vi "StopMotion.vi"(8 "error in (no error)":errorcluster, 11 "UI ExecutionCtrls in":refnum<class "UI ExecutionCtrls.lvclass">) -> (0 "error out":errorcluster, 3 "UI ExecutionCtrls out":refnum<class "UI ExecutionCtrls.lvclass">)   [LabVIEW 2018, in "UI ExecutionCtrls.lvclass"]
uses:
  UI ExecutionCtrls.lvclass
  UI ExecutionCtrls.lvclass/UI ExecutionCtrls.ctl
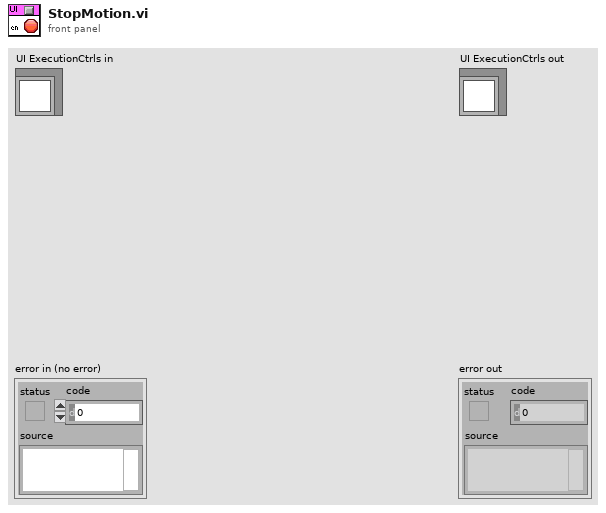
[diagram p1: front panel]
types:
  T1 = enum8{"Enabled", "Disabled", "Disabled and Grayed Out"}
  T2 = typedef "MotionExecutionCtrlRefs.ctl" = cluster{"MoveAllAbsolute":refnum<vi>, "Move to Pos.":refnum<vi>, "HomeAll":refnum<vi>, "FindHomeAll":refnum<vi>, "X Jog Pos.":refnum<vi>, "X Jog Neg.":refnum<vi>, "Y Jog Pos.":refnum<vi>, "Y Jog Neg. ":refnum<vi>, "Z Jog Pos.":refnum<vi>, "Z Jog Neg.":refnum<vi>, "T Jog Pos.":refnum<vi>, "T Jog Neg.":refnum<vi>, "X Home Button":refnum<vi>, "Y Home Button":refnum<vi>, "Z Home Button":refnum<vi>, "T Home Button":refnum<vi>}
  T3 = typedef "mmWaveMotionCrtlRefs.ctl" = cluster{"BS3 Jog Neg. 2":refnum<vi>, "BS3 Jog Pos. 2":refnum<vi>, "BS3 Home Button 2":refnum<vi>, "BS4 Jog Neg. 2":refnum<vi>, "BS4 Jog Pos. 2":refnum<vi>, "BS4 Home Button 2":refnum<vi>, "RT2 Jog Neg. 2":refnum<vi>, "RT2 Jog Pos. 2":refnum<vi>, "RT2 Home Button 2":refnum<vi>}
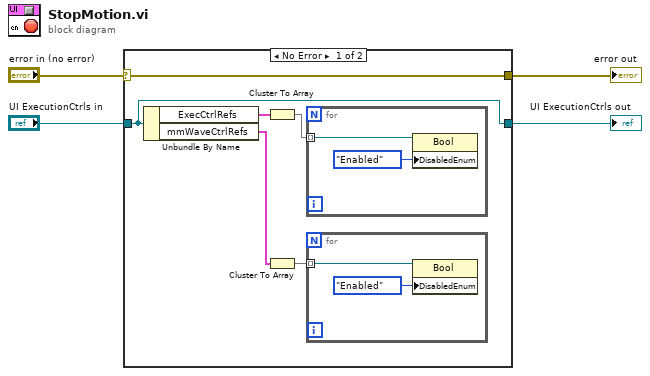
[diagram p0: block diagram]
diagram:
  n1 = case shown="No Error" "error in (no error)" {
    selector: "error in (no error)" -> [w10 w16]
    tunnel: [w10 w16] -> w1
    tunnel: [w7 w15] -> w2
    tunnel: "UI ExecutionCtrls in" -> [w7 w15]
    frame No Error {
      n2 = Unbundle By Name(w7) -> ("ExecCtrlRefs"=w8:T2, "mmWaveCtrlRefs"=w5:T3)
      n3 = Cluster To Array(cluster=w8) -> (array=w9:refnum<vi>[])
      n4 = Cluster To Array(cluster=w5) -> (array=w6:refnum<vi>[])
      n5 = for {
        tunnel: w9 -> [w14] mode=indexing
        n6 = property class="Bool"(reference=w14, "DisabledEnum"=T1."Enabled" ("Disabled")) -> ()  [unwired: 1 in, 2 out]
      }
      n7 = for {
        tunnel: w6 -> [w12] mode=indexing
        n8 = property class="Bool"(reference=w12, "DisabledEnum"=T1."Enabled" ("Disabled")) -> ()  [unwired: 1 in, 2 out]
      }
    }
    frame Error {
    }
  }
  "error out" <- w1
  "UI ExecutionCtrls out" <- w2
